vi "Remove Null Characters.vi"(4 "String":string) -> (1 "string":string)   [LabVIEW 2015]
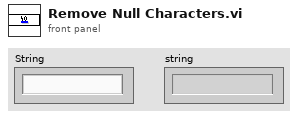
[diagram p1: front panel]
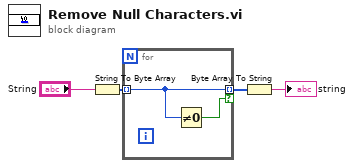
[diagram p0: block diagram]
diagram:
  n1 = String To Byte Array(string="String") -> (unsigned byte array=w1:u8[])
  n2 = for {
    tunnel: w1 -> [w5] mode=indexing
    tunnel: [w5] -> w2 mode=indexing if=w6
    n3 = Not Equal To 0?(x=w5) -> (x != 0?=w6:bool)
  }
  n4 = Byte Array To String(unsigned byte array=w2) -> (string=→"string":string)
